vi "SVT THD+N (Frequency) (1 Ch).vi"(0 "complex spectrum":T7={"complex spectrum response"={"f0"=0.0, "df"=1.0, "complex spectrum"=[]}, "spectrum info"={"channel name"="", "description"="", "x-axis units"=0, "spectral info"={"spectrum type"=enum."Power [Magnitude^2]", "linear/dB"=enum."linear", "window"=0, "window size"=0, "FFT size"=0}, "engineering units"=0, "custom label"="", "dB reference [EU]"=0.0, "peak units"=enum."rms", "weighting filter"=0, "spectral density?"=FALSE, "unit label"="", "spectrum skewed?"=FALSE, "complimentary spectrum units"=enum."none"}} {"spectrum info"."x-axis units" items=["Time (s)"=0, "Frequency-CB (Hz)"=1, "Frequency-CPB (Hz)"=1248, "Frequency-Arbitrary (Hz)"=2357, "Quefrency (s)"=2, "Revolutions (rev)"=3, "Order"=4, "Speed (RPM)"=11, "Speed (rad/s)"=21, "Index"=65535]; "spectrum info"."weighting filter" items=["Linear", "A-weighting", "B-weighting", "C-weighting", "ITU-R 468-4", "Dolby", "CCITT", "C-message", "Wb", "Wc", "Wd", "We", "Wf", "Wh", "Wj", "Wk", "Wm", "AES17 20 kHz lowpass", "AES17 40 kHz lowpass", "AES17 20 kHz highpass", "AES17 40 kHz highpass"]; "spectrum info"."dB reference [EU]" format="%.2f"; "spectrum info"."engineering units" items=["custom..."=0, "V"=1, "A"=21, "C"=30, "pC"=31, "s"=32, "-"=29, "Pa"=2, "N"=20, "g"=3, "m/s^2"=4, "m/s"=5, "m"=6, "mm/s"=12, "mm"=13, "micron/s"=14, "micron"=15, "in/s^2"=7, "in/s"=8, "in"=9, "mil/s"=10, "mil"=11, "rad/s^2"=16, "rad/s"=17, "rad"=18, "deg/s^2"=26, "deg/s"=27, "deg"=28, "RPM"=22, "cycle/s^2"=23, "Hz"=24, "cycle"=25, "strain"=19]; "spectrum info"."spectral info"."window" items=["None "=0, "Hanning"=1, "Hamming"=2, "Blackman-Harris"=3, "Exact Blackman"=4, "Blackman"=5, "Flat Top"=6, "4 Term B-Harris "=7, "7 Term B-Harris"=8, "Low Sidelobe"=9, "Force - Exponential"=10, "Gaussian"=62]; "complex spectrum response"."complex spectrum" format="%.2f"; "complex spectrum response"."df" format="%.2f"; "complex spectrum response"."f0" format="%.2f"}, 2 "frequency range":T9={"start frequency"=-1.0, "stop frequency"=-1.0} {"stop frequency" format="%.2f"; "start frequency" format="%.2f"}, 3 "advanced span [Hz]":dbl=-1.0 format="%.2f", 5 "error in (no error)":errorcluster, 6 "desired units":T10, 9 "expected fundamental frequency [Hz]":dbl=-1.0 format="%.2f") -> (11 "detected fundamental\nfrequency [Hz]":dbl format="%.2f", 12 "unit labels":T8, 13 "detected fundamental\namplitude":dbl format="%.2f", 14 "dup complex spectrum":T7={"complex spectrum response"={"f0"=0.0, "df"=1.0, "complex spectrum"=[]}, "spectrum info"={"channel name"="", "description"="", "x-axis units"=0, "spectral info"={"spectrum type"=enum."Power [Magnitude^2]", "linear/dB"=enum."linear", "window"=0, "window size"=0, "FFT size"=0}, "engineering units"=0, "custom label"="", "dB reference [EU]"=0.0, "peak units"=enum."rms", "weighting filter"=0, "spectral density?"=FALSE, "unit label"="", "spectrum skewed?"=FALSE, "complimentary spectrum units"=enum."none"}} {"spectrum info"."x-axis units" items=["Time (s)"=0, "Frequency-CB (Hz)"=1, "Frequency-CPB (Hz)"=1248, "Frequency-Arbitrary (Hz)"=2357, "Quefrency (s)"=2, "Revolutions (rev)"=3, "Order"=4, "Speed (RPM)"=11, "Speed (rad/s)"=21, "Index"=65535]; "spectrum info"."weighting filter" items=["Linear", "A-weighting", "B-weighting", "C-weighting", "ITU-R 468-4", "Dolby", "CCITT", "C-message", "Wb", "Wc", "Wd", "We", "Wf", "Wh", "Wj", "Wk", "Wm", "AES17 20 kHz lowpass", "AES17 40 kHz lowpass", "AES17 20 kHz highpass", "AES17 40 kHz highpass"]; "spectrum info"."dB reference [EU]" format="%.2f"; "spectrum info"."engineering units" items=["custom..."=0, "V"=1, "A"=21, "C"=30, "pC"=31, "s"=32, "-"=29, "Pa"=2, "N"=20, "g"=3, "m/s^2"=4, "m/s"=5, "m"=6, "mm/s"=12, "mm"=13, "micron/s"=14, "micron"=15, "in/s^2"=7, "in/s"=8, "in"=9, "mil/s"=10, "mil"=11, "rad/s^2"=16, "rad/s"=17, "rad"=18, "deg/s^2"=26, "deg/s"=27, "deg"=28, "RPM"=22, "cycle/s^2"=23, "Hz"=24, "cycle"=25, "strain"=19]; "spectrum info"."spectral info"."window" items=["None "=0, "Hanning"=1, "Hamming"=2, "Blackman-Harris"=3, "Exact Blackman"=4, "Blackman"=5, "Flat Top"=6, "4 Term B-Harris "=7, "7 Term B-Harris"=8, "Low Sidelobe"=9, "Force - Exponential"=10, "Gaussian"=62]; "complex spectrum response"."complex spectrum" format="%.2f"; "complex spectrum response"."df" format="%.2f"; "complex spectrum response"."f0" format="%.2f"}, 16 "THD+N":dbl format="%.2f", 19 "error out":errorcluster)   [LabVIEW 2017, in "SoundVib_Distortion.lvlib"]
doc: "Performs a total harmonic distortion plus noise (THD+N) analysis, including measuring the fundamental tone, and returns the detected fundamental frequency, detected fundamental amplitude, and THD+N. Signal in noise and distortion (SINAD) is the negative of THD+N in dB. Wire data to the<B> scaled signal [EU]</B> input to determine the polymorphic instance to use or manually select the instance.\n\nThe following formula calculates THD+N:\n\nTHD+N = sqrt(H^2 + N^2) / sqrt(F^2 + N^2 + H^2)\n\nwhere H is the harmonic RMS level, N is the noise RMS level, and F is the fundamental tone RMS level."
uses:
  <vilib>/addons/Sound and Vibration/svt_Distortion/SoundVib_Distortion.lvlib
  <vilib>/addons/_NISVFA/_Shared subVIs/Controls/svc_Spectrum Info.ctl
  <vilib>/addons/_NISVFA/_Shared subVIs/Controls/svc_X-Axis Units.ctl
  <vilib>/addons/_NISVFA/_Shared subVIs/Controls/svc_Spectrum Type.ctl
  <vilib>/addons/_NISVFA/_Shared subVIs/Controls/svc_Engineering Units Text Ring.ctl
  <vilib>/addons/_NISVFA/_Shared subVIs/Controls/svc_Weighting Filter Text Ring.ctl
  <vilib>/addons/_NISVFA/_Shared subVIs/Controls/svc_Complimentary Spectrum Units.ctl
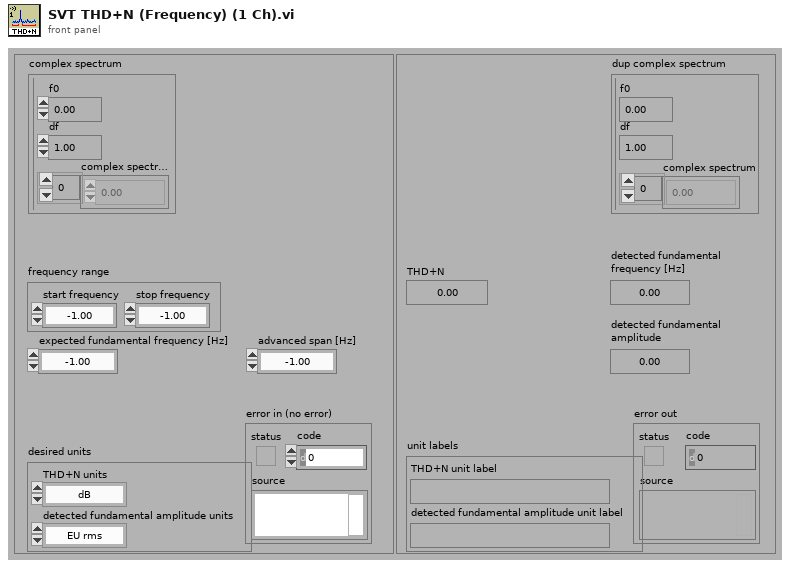
[diagram p1: front panel]
types:
  T1 = typedef "svc_Spectrum Info.ctl" = cluster{"channel name":string, "description":string, "x-axis units":T2, "spectral info":cluster{"spectrum type":T3, "linear/dB":enum16{"linear", "dB"}, "window":u16, "window size":i32, "FFT size":i32}, "engineering units":T4, "custom label":string, "dB reference [EU]":dbl, "peak units":enum16{"rms", "peak", "peak-peak"}, "weighting filter":T5, "spectral density?":bool, "unit label":string, "spectrum skewed?":bool, "complimentary spectrum units":T6}
  T2 = typedef "svc_X-Axis Units.ctl" = u16
  T3 = typedef "svc_Spectrum Type.ctl" = enum16{"FFT Spectrum [complex]", "Amplitude [Magnitude]", "Power [Magnitude^2]", "Cross Spectrum [complex]", "Frequency Response [Complex]"}
  T4 = typedef "svc_Engineering Units Text Ring.ctl" = u16
  T5 = typedef "svc_Weighting Filter Text Ring.ctl" = u16
  T6 = typedef "svc_Complimentary Spectrum Units.ctl" = enum16{"none", "radians", "degrees", "cycles", "imaginary"}
  T7 = cluster{"complex spectrum response":cluster{"f0":dbl, "df":dbl, "complex spectrum":cdb[]}, "spectrum info":T1}
  T8 = cluster{"THD+N unit label":string, "detected fundamental amplitude unit label":string}
  T9 = cluster{"start frequency":dbl, "stop frequency":dbl}
  T10 = cluster{"THD+N units":enum16{"dB", "linear ratio", "%"}, "detected fundamental amplitude units":enum16{"EU rms", "EU peak", "EU peak-peak"}}
  T11 = cluster{"unit label":string, "unit label":string}
  T12 = cluster{"SINAD [ratio]":dbl, "THD+N [ratio]":dbl, "THD":dbl}
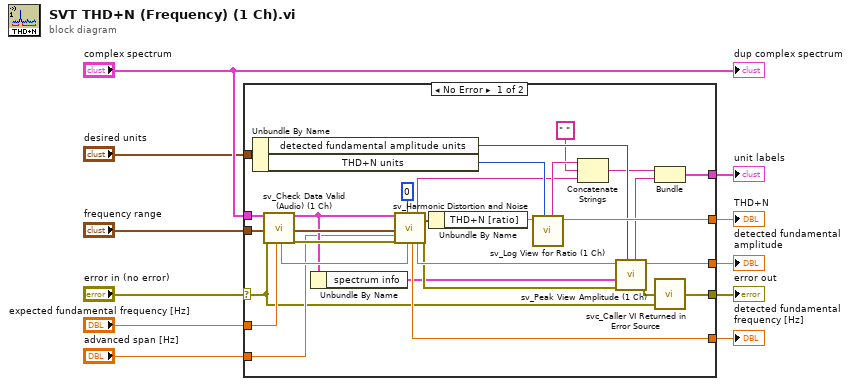
[diagram p0: block diagram]
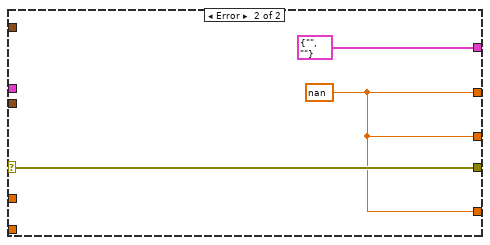
[diagram p2: hidden frame]
diagram:
  n1 = case shown="No Error" "error in (no error)" {
    selector: "error in (no error)" -> [w15 w43]
    tunnel: "complex spectrum" -> [w24 _]
    tunnel: "expected fundamental frequency [Hz]" -> [w26 _]
    tunnel: [w39 w43] -> w9
    tunnel: [w35 w42] -> w8
    tunnel: [w40 w42] -> w7
    tunnel: [w37 w42] -> w5
    tunnel: "frequency range" -> [w21 _]
    tunnel: "desired units" -> [w36 _]
    tunnel: [w31 T11 {"unit label"="", "unit label"=""}] -> w2
    tunnel: "advanced span [Hz]" -> [w16 _]
    frame No Error {
      n2 = Unbundle By Name(w36) -> ("detected fundamental amplitude units"=w32:enum16{"EU rms", "EU peak", "EU peak-peak"}, "THD+N units"=w34:enum16{"dB", "linear ratio", "%"})
      n3 = call <vilib>:"sv_Check Data Valid (Audio) (1 Ch).vi"("complex spectrum"=w24, "frequency range in"=w21, "error in (no error)"=w15, "expected fundamental frequency [Hz]"=w26) -> ("dup expected fundamental frequency [Hz]"=w25:dbl, "complex spectrum"=w18:T7, "frequency range out"=w22:T9, "error out"=w23:errorcluster)  [unwired: 8 in, 4 out]
      n4 = Unbundle By Name(w18) -> ("spectrum info"=w17:T1)
      n5 = call <vilib>:"sv_Harmonic Distortion and Noise.vi"("complex spectrum"=w18, "frequency range"=w22, "advanced span [Hz]"=w16, "error in"=w23, "maximum harmonic"=0, "approx. fund. freq. (optional)"=w25) -> ("detected fundamental frequency"=w40:dbl, "frequency range string"=w28:string, "detected amplitude"=w38:dbl, "distortion measurements"=w13:T12, "error out"=w19:errorcluster)  [unwired: 6 in, 3 out]
      n6 = Unbundle By Name(w13) -> ("THD+N [ratio]"=w12:dbl)
      n7 = call <vilib>:"sv_Log View for Ratio (1 Ch).vi"("ratio units"=w34, "linear ratio"=w12) -> ("converted ratio"=w35:dbl, "unit label"=w30:string)  [unwired: 7 in, 1 out]
      n8 = Concatenate Strings(w30, " " ("string"), w28) -> (w29:string)
      n9 = call <vilib>:"sv_Peak View Amplitude (1 Ch).vi"("peak units"=w32, "error in (no error)"=w19, "spectrum info"=w17, "peak amplitude [EU pk]"=w38) -> ("error out"=w20:errorcluster, "converted peak amplitude"=w37:dbl, "unit label"=w33:string)  [unwired: 5 in]
      n10 = Bundle(w29, "unit label"=w33) -> (w31:cluster{string, "unit label":string})  [unwired: 1 in]
      n11 = call <vilib>:"svc_Caller VI Returned in Error Source.vi"("warning input to caller"=w15, "error in (no error)"=w20) -> ("error out"=w39:errorcluster)  [unwired: 3 in]
    }
    frame Error {
      w42 = nan ("SINAD")
    }
  }
  "error out" <- w9
  "detected fundamental\nfrequency [Hz]" <- w7
  "THD+N" <- w8
  "unit labels" <- w2
  "detected fundamental\namplitude" <- w5
  "dup complex spectrum" <- "complex spectrum"
